vi "Checkout.vi"(5 "RobRef":dbl[](array[numeric]), 6 "Array":string, 7 "CamRef":dbl[](array[numeric]), 8 "camera y":dbl, 9 "camera x":dbl, 11 "RobSnap":dbl[](array[numeric])) -> (1 "robot y":dbl, 2 "robot x":dbl)   [LabVIEW 2016]
panel:
  # "标定结果验证"
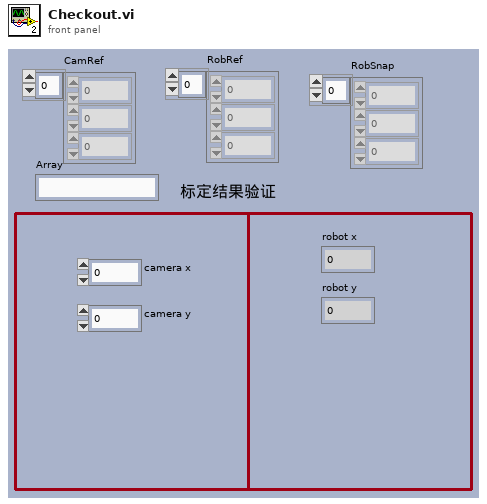
[diagram p1: front panel]
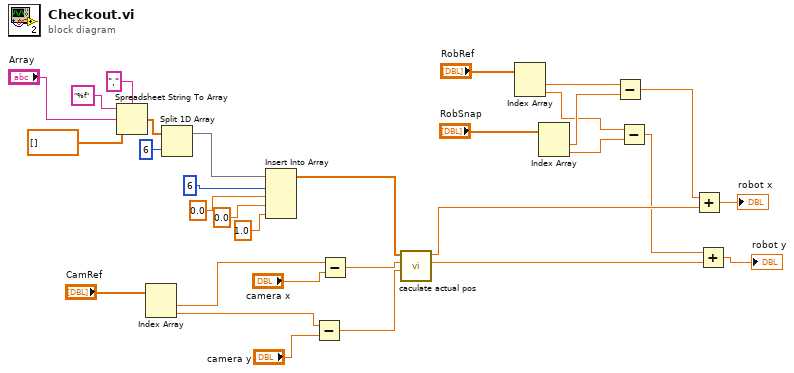
[diagram p0: block diagram]
diagram:
  n1 = Spreadsheet String To Array(delimiter (Tab)=",", format string="%f" ("spreadsheet string"), spreadsheet string="Array", array type (2D Dbl)=dbl[] []) -> (array=w25:dbl[])
  n2 = Index Array(array="CamRef") -> (element #1=w3:dbl, element #2=w1:dbl)  [unwired: 2 in]
  n3 = Split 1D Array(array=w25, index=6) -> (first subarray=w30:dbl[])  [unwired: 1 out]
  n4 = Insert Into Array(array=w30, index=6, new element #1=0.0 ("new element/subarray"), new element #2=0.0 ("new element/subarray"), new element #3=1.0 ("new element/subarray")) -> (w31:dbl[])
  n5 = Subtract(x=w1, y="camera y") -> (x-y=w17:dbl)
  n6 = Subtract(x=w3, y="camera x") -> (x-y=w18:dbl)
  n7 = call "caculate actual pos.vi"("camera y"=w17, "camera x"=w18, "Array"=w31) -> ("robot y"=w10:dbl, "robot x"=w13:dbl)  [unwired: 7 in]
  n8 = Index Array(array="RobRef") -> (element #1=w8:dbl, element #2=w6:dbl)  [unwired: 2 in]
  n9 = Index Array(array="RobSnap") -> (element #1=w7:dbl, element #2=w5:dbl)  [unwired: 2 in]
  n10 = Subtract(x=w8, y=w7) -> (x-y=w14:dbl)
  n11 = Subtract(x=w6, y=w5) -> (x-y=w11:dbl)
  n12 = Add(x=w14, y=w13) -> (x+y=→"robot x":dbl)
  n13 = Add(x=w11, y=w10) -> (x+y=→"robot y":dbl)
